vi "Motion_Wait for Loader Home.vi"(8 "error in":errorcluster, 10 "timeout (60s)":dbl[unit]=60.0 caption="Time Target (s)" format="%.1f", 11 "TCP refnum":refnum<k5>) -> (0 "error out":errorcluster, 1 "Loader At Home":bool, 2 "elapsed time":dbl[unit]=nan format="%.1f", 3 "TCP refnum dup":refnum<k5>, 4 "timeout error":bool, 5 "done":bool)   [LabVIEW 2010]
panel:
  in  "poll interval (0.1s)":dbl[unit]=0.1
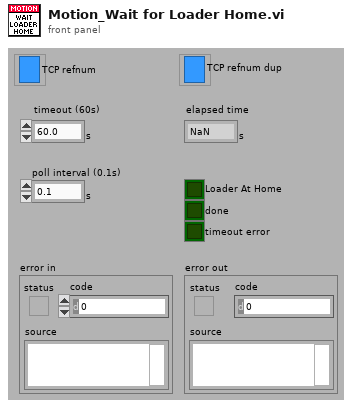
[diagram p1: front panel]
types:
  T1 = cluster{"Loader Enabled":bool, "Loader Alarm ":bool, "Loader Warning":bool, "Loader At Connect":bool, "Loader At Load":bool, "Loader Connect Aborted":bool, "Loader Connect Error":bool, "Loader Connecting":bool, "Loader Control Alarm":bool, "Loader At Home":bool, "Loader Home Error":bool, "Loader Home Aborted":bool, "Loader Homing":bool, "Loader Load Aborted":bool, "Loader Load Error":bool, "Loader Loading":bool, "Loader Stop Aborted":bool, "Loader Stop Error":bool, "Loader Stopped":bool, "Loader Stopping":bool, "Loader General Alarm":bool, "Motion Alarm":bool, "Loader Home Required":bool}
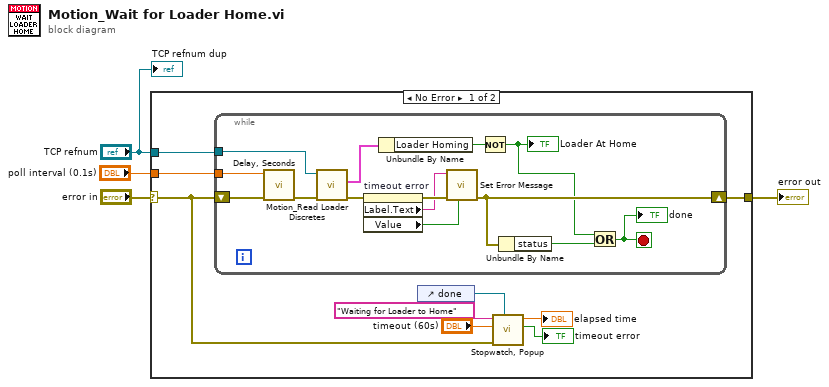
[diagram p0: block diagram]
diagram:
  n1 = case shown="No Error" "error in" {
    selector: "error in" -> [w6 w28]
    tunnel: "TCP refnum" -> [w8 _]
    tunnel: [w7 w28] -> w4
    tunnel: "poll interval (0.1s)" -> [w5 _]
    frame No Error {
      n2 = while {
        tunnel: w8 -> [w17]
        shift-right: [w23] -> w7
        shift-left: w6 -> [w27]
        tunnel: w5 -> [w21]
        stop <- w18 stop-if-true
        n3 = call "Delay, Seconds.vi"("error in"=w27, "delay"=w21) -> ("error out"=w15:errorcluster)  [unwired: 5 in, 1 out]
        n4 = call "Motion_Read Loader Discretes.vi"("error in (no error)"=w15, "TCP Connection Refnum in"=w17) -> ("error out"=w14:errorcluster, "Loader Discretes"=w16:T1)  [unwired: 7 in, 1 out]
        n5 = property on="timeout error" class="Bool (strict)"(error in=w14) -> (error out=w26:errorcluster, "Label.Text"=w24:string, "Value"=w25:bool)  [unwired: 1 in, 1 out]
        n6 = Unbundle By Name(w16) -> ("Loader Homing"=w20:bool)
        n7 = call "Set Error Message.vi"("enable (T)"=w25, "error in"=w26, "message"=w24) -> ("error out"=w23:errorcluster)  [unwired: 5 in]
        n8 = Not(x=w20) -> (.not. x?=w19:bool)
        "Loader At Home" <- w19
        n9 = Unbundle By Name(w23) -> ("status"=w22:bool)
        n10 = Or(x=w19, y=w22) -> (x .or. y?=w18:bool)
        "done" <- w18
      }
      n11 = control-ref of="done"() -> (w12:refnum<vi>)
      n12 = call "Stopwatch, Popup.vi"("Stop (Bool) Refnum"=w12, "error in (no error)"=w6, "Time Target"="timeout (60s)", "Front Panel Window:Title"="Waiting for Loader to Home") -> ("Time has Elapsed"=→"timeout error":bool, "Elapsed Time (Knob)"=→"elapsed time":dbl[unit])  [unwired: 5 in, 1 out]
    }
    frame Error {
    }
  }
  "error out" <- w4
  "TCP refnum dup" <- "TCP refnum"
